vi "Read Page Orientaion V2.vi"(0 "PDF Report IN":refnum<class "PDF Report Class.lvclass">, 5 "PdfReader ref":refnum<k24>, 7 "PdfReader page number":i32=-1, 9 "Page (points)":T2={"Start at page"=1, "Page Size"=0, "Orientation"=enum."Landscape", "widht"=792.0, "height"=72.0, "Margin left"=72.0, "Margin right"=72.0, "Margin top"=72.0, "Margin bottom"=72.0, "X0"=0.0, "X1"=612.0, "Y0"=0.0, "Y1"=792.0} {"Page Size" items=["Custom", "LETTER", "NOTE", "LEGAL", "TABLOID", "EXECUTIVE", "POSTCARD", "A0", "A1", "A2", "A3", "A4", "A5", "A6", "A7", "A8", "A9", "A10", "B0", "B1", "B2", "B3", "B4", "B5", "B6", "B7", "B8", "B9", "B10", "ARCH_E", "ARCH_D", "ARCH_C", "ARCH_B", "ARCH_A", "FLSA", "FLSE", "HALFLETTER", "_11X17", "ID_1", "ID_2", "ID_3", "LEDGER", "CROWN_QUARTO", "LARGE_CROWN_QUARTO", "DEMY_QUARTO", "ROYAL_QUARTO", "CROWN_OCTAVO", "LARGE_CROWN_OCTAVO", "DEMY_OCTAVO", "ROYAL_OCTAVO", "SMALL_PAPERBACK", "PENGUIN_SMALL_PAPERBACK", "PENGUIN_LARGE_PAPERBACK"]}, 11 "error in (no error)":errorcluster) -> (4 "PDF Report OUT":refnum<class "PDF Report Class.lvclass">, 6 "PdfReader ref duplicate":refnum<k24>, 10 "Orientation":T1, 15 "error out":errorcluster)   [LabVIEW 2019, in "Exaprom PDF.lvlib"]
doc: "Version 1.1\nDeveloped by Jean-Marc Simard\nCopyright © 2012, Exaprom Inc.\nAll rights reserved.\nLicense: BSD\n\nWith iTextSharp 4.1.6 (http://itextsharp.sourceforge.net)\nunder Mozilla Public License Version 1.1\n(http://www.mozilla.org/MPL/MPL-1.1.html)"
uses:
  C:/work/niobrara_lv/labview pdf writer fixing/DLL/itextsharp.dll
  DLL/itextsharp.dll
  Controls/Page Controls/Page dimensions.ctl
  Controls/Page Controls/Page Orientation.ctl
  LV Class/PDF Report Class/PDF Report Class.lvclass
  Controls/Page Controls/Page setup.ctl
  Controls/Page Controls/Page Layout Custom.ctl
  Controls/Page Controls/Page margins.ctl
  Exaprom PDF.lvlib
  Controls/Page Controls/Page size.ctl
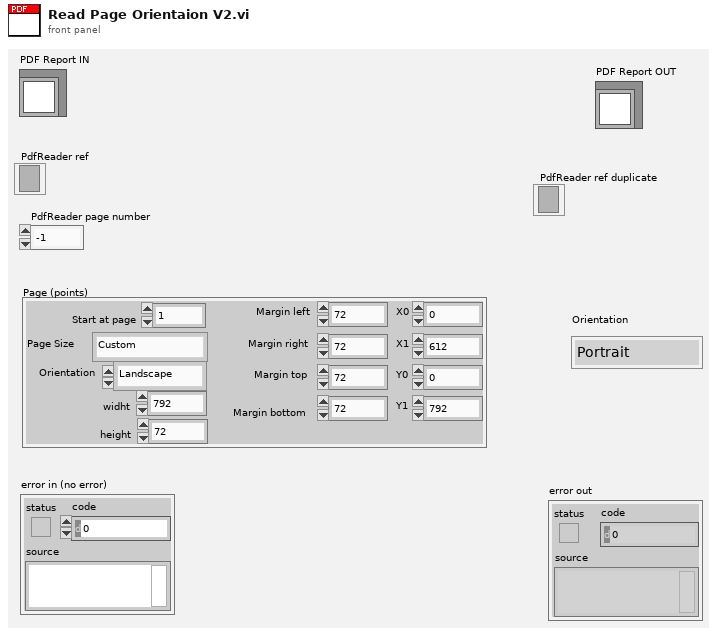
[diagram p1: front panel]
types:
  T1 = typedef "Exaprom PDF.lvlib/Page Orientation.ctl" = enum16{"Portrait", "Landscape"}
  T2 = typedef "Exaprom PDF.lvlib/Page dimensions.ctl" = cluster{"Start at page":i32, "Page Size":T3, "Orientation":T1, "widht":sgl, "height":sgl, "Margin left":sgl, "Margin right":sgl, "Margin top":sgl, "Margin bottom":sgl, "X0":sgl, "X1":sgl, "Y0":sgl, "Y1":sgl}
  T3 = typedef "Exaprom PDF.lvlib/Page size.ctl" = i32
  T4 = typedef "Exaprom PDF.lvlib/Page setup.ctl" = cluster{"Page Size":T3, "Orientation":T1, "Custom Size":T5, "Margins":T6}
  T5 = typedef "Exaprom PDF.lvlib/Page Layout Custom.ctl" = cluster{"Width":sgl, "Height":sgl}
  T6 = typedef "Exaprom PDF.lvlib/Page margins.ctl" = cluster{"Left":sgl, "Right":sgl, "Top":sgl, "Bottom":sgl}
  T7 = typedef "Exaprom PDF.lvlib/Unit.ctl" = enum16{"inch", "mm"}
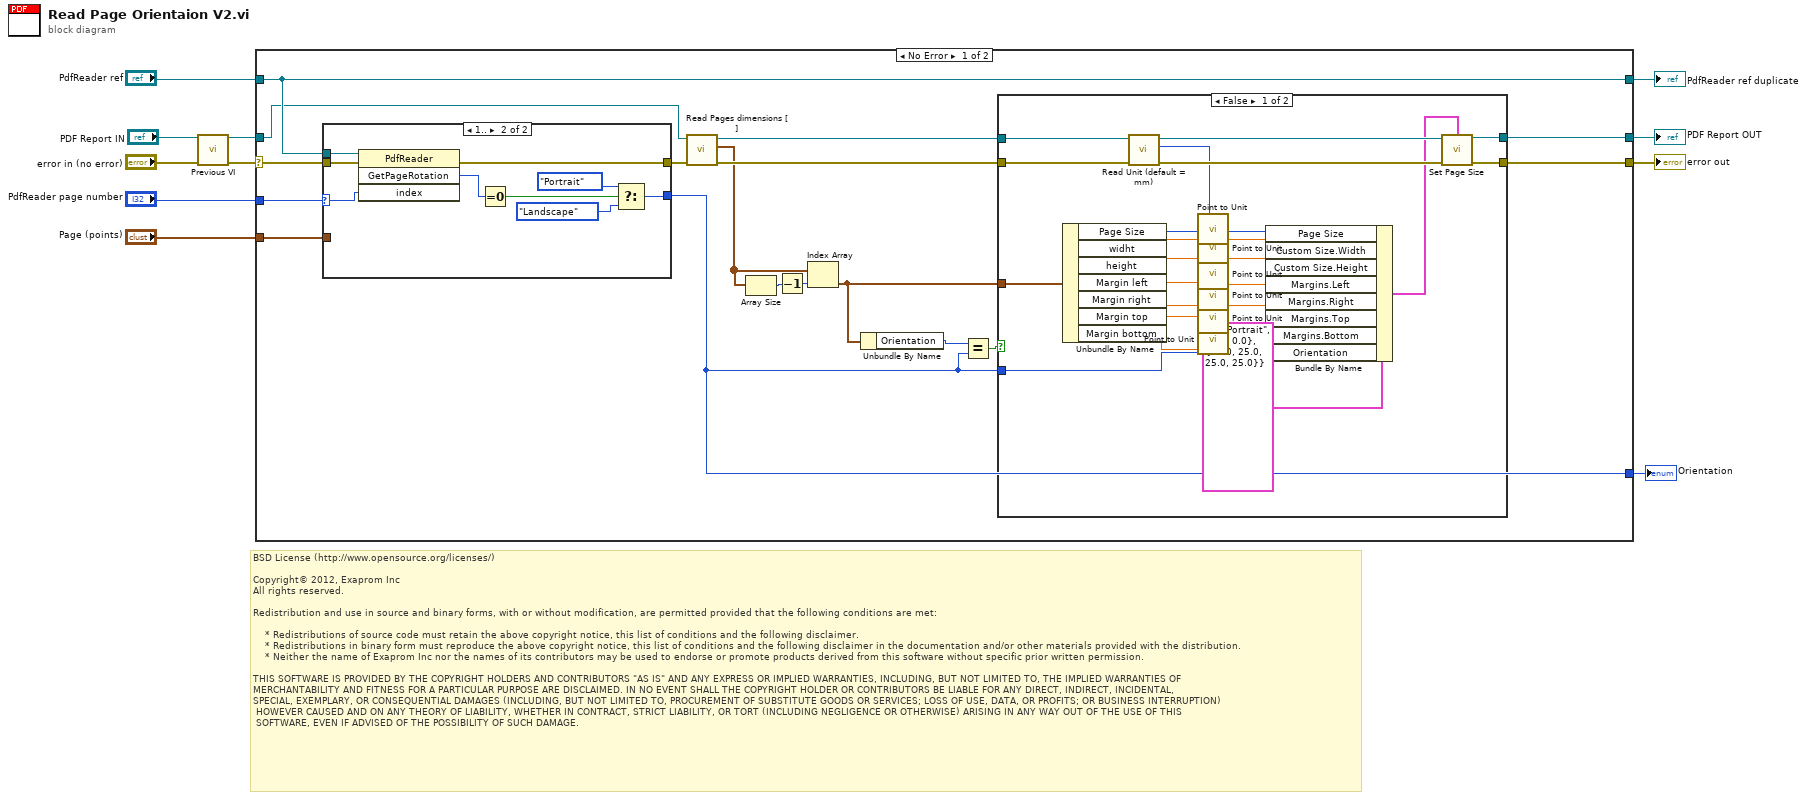
[diagram p0: block diagram]
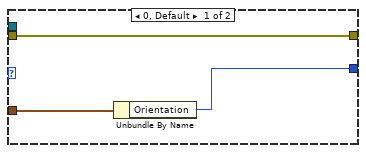
[diagram p2: hidden frame]
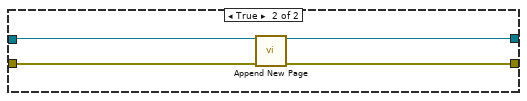
[diagram p3: hidden frame]
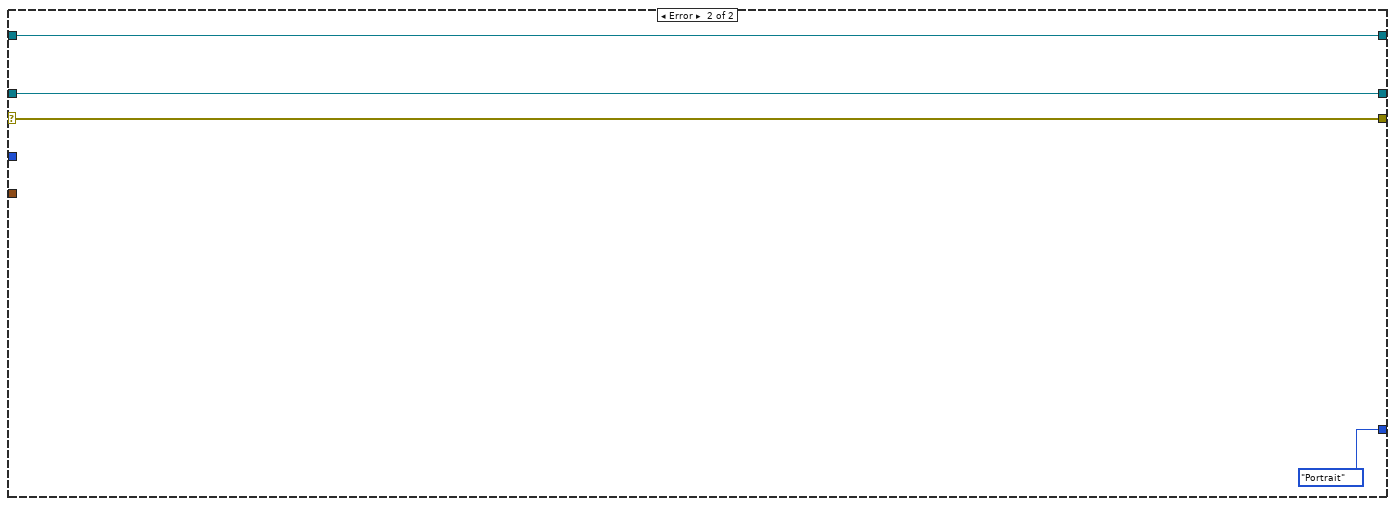
[diagram p4: hidden frame]
diagram:
  # "BSD License (http://www.opensource.org/licenses/)\n\nCopyright© 2012, Exaprom Inc\nAll rights reserved.\n\nRedistribution and use in source and binary forms, with or without modification, are permitted provided that the following conditions are met:\n\n    * Redistributions of source code must retain the above copyright notice, this list of conditions and the following disclaimer.\n    * Redistributions in binary form must reproduce the above copyright notice, this list of conditions and the following disclaimer in the documentation and/or other materials provided with the distribution.\n    * Neither the name of Exaprom Inc nor the names of its contributors may be used to endorse or promote products derived from this software without specific prior written permission.\n\nTHIS SOFTWARE IS PROVIDED BY THE COPYRIGHT HOLDERS AND CONTRIBUTORS \"AS IS\" AND ANY EXPRESS OR IMPLIED WARRANTIES, INCLUDING, BUT NOT LIMITED TO, THE IMPLIED WARRANTIES OF \nMERCHANTABILITY AND FITNESS FOR A PARTICULAR PURPOSE ARE DISCLAIMED. IN NO EVENT SHALL THE COPYRIGHT HOLDER OR CONTRIBUTORS BE LIABLE FOR ANY DIRECT, INDIRECT, INCIDENTAL,\nSPECIAL, EXEMPLARY, OR CONSEQUENTIAL DAMAGES (INCLUDING, BUT NOT LIMITED TO, PROCUREMENT OF SUBSTITUTE GOODS OR SERVICES; LOSS OF USE, DATA, OR PROFITS; OR BUSINESS INTERRUPTION)\n HOWEVER CAUSED AND ON ANY THEORY OF LIABILITY, WHETHER IN CONTRACT, STRICT LIABILITY, OR TORT (INCLUDING NEGLIGENCE OR OTHERWISE) ARISING IN ANY WAY OUT OF THE USE OF THIS\n SOFTWARE, EVEN IF ADVISED OF THE POSSIBILITY OF SUCH DAMAGE."
  n1 = call "Previous VI.vi"("PDF Report IN"="PDF Report IN", "error in (no error)"="error in (no error)") -> ("PDF Report OUT"=w5:refnum<class "PDF Report Class.lvclass">, "error out"=w2:errorcluster)  [unwired: 12 out]
  n2 = case shown="No Error" w2 {
    selector: w2 -> [w26 w72]
    tunnel: [w23 w72] -> w11
    tunnel: [w16 w71] -> w10
    tunnel: "PdfReader page number" -> [w14 _]
    tunnel: "PdfReader ref" -> [w16 w71]
    tunnel: "Page (points)" -> [w13 _]
    tunnel: w5 -> [w15 w70]
    tunnel: [w22 w70] -> w6
    tunnel: [w12 Page_Orientation."Portrait" ("Orientation")] -> w1
    frame No Error {
      n3 = case shown="1.." w14 {
        selector: w14 -> [_ w37]
        tunnel: w26 -> [w31 w40]
        tunnel: [w31 w39] -> w24
        tunnel: w16 -> [_ w38]
        tunnel: [w29 w32] -> w12
        tunnel: w13 -> [w30 _]
        frame 0, Default {
          n4 = Unbundle By Name(w30) -> ("Orientation"=w29:T1)
        }
        frame 1.. {
          n5 = invoke class="PdfReader" method="GetPageRotation"(reference=w38, error in=w40, "index"=w37) -> (error out=w39:errorcluster, "GetPageRotation"=w33:i32)  [unwired: 1 in, 2 out]
          n6 = Equal To 0?(x=w33) -> (x = 0?=w36:bool)
          n7 = Select(t=Page_Orientation."Portrait" ("Orientation"), s=w36, f=Page_Orientation."Landscape" ("Orientation")) -> (s? t:f=w32:T1)
        }
      }
      n8 = call-dynamic "Read Pages dimensions [ ].vi"("error in (no error)"=w24, "PDF Report Class in"=w15) -> ("error out"=w21:errorcluster, "Pages dimensions [ ]"=w18:T2[], "PDF Report Class out"=w20:refnum<class "PDF Report Class.lvclass">)  [unwired: 6 in, 1 out]
      n9 = Array Size(array=w18) -> (size(s)=w28:i32)
      n10 = Decrement(x=w28) -> (x-1=w27:i32)
      n11 = Index Array(array=w18, index=w27) -> (element=w17:T2)
      n12 = Unbundle By Name(w17) -> ("Orientation"=w19:T1)
      n13 = Equal?(x=w19, y=w12) -> (x = y?=w25:bool)
      n14 = case shown="False" w25 {
        tunnel: w21 -> [w64 w68]
        tunnel: [w63 w67] -> w23
        tunnel: [w62 w65] -> w22
        tunnel: w20 -> [w60 w66]
        tunnel: w17 -> [w58 _]
        tunnel: w12 -> [w41 _]
        frame False {
          n15 = Unbundle By Name(w58) -> ("Page Size"=w43:T3, "widht"=w56:sgl, "height"=w52:sgl, "Margin left"=w54:sgl, "Margin right"=w48:sgl, "Margin top"=w53:sgl, "Margin bottom"=w45:sgl)
          n16 = call-dynamic "Read Unit (default = mm).vi"("error in (no error)"=w64, "PDF Report Class in"=w60) -> ("error out"=w61:errorcluster, "Unit (default = mm)"=w44:T7, "PDF Report Class out"=w59:refnum<class "PDF Report Class.lvclass">)  [unwired: 7 in]
          n17 = call "Point to Unit.vi"("X point"=w56, "Unit (default = mm)"=w44) -> ("X unit"=w55:sgl)  [unwired: 7 in]
          n18 = call "Point to Unit.vi"("X point"=w52, "Unit (default = mm)"=w44) -> ("X unit"=w51:sgl)  [unwired: 7 in]
          n19 = call "Point to Unit.vi"("X point"=w54, "Unit (default = mm)"=w44) -> ("X unit"=w50:sgl)  [unwired: 7 in]
          n20 = call "Point to Unit.vi"("X point"=w48, "Unit (default = mm)"=w44) -> ("X unit"=w49:sgl)  [unwired: 7 in]
          n21 = call "Point to Unit.vi"("X point"=w53, "Unit (default = mm)"=w44) -> ("X unit"=w47:sgl)  [unwired: 7 in]
          n22 = call "Point to Unit.vi"("X point"=w45, "Unit (default = mm)"=w44) -> ("X unit"=w46:sgl)  [unwired: 7 in]
          n23 = Bundle By Name(cluster=T4 {"Page Size"=1, "Orientation"=enum."Portrait", "Custom Size"={"Width"=0.0, "Height"=0.0}, "Margins"={"Left"=25.0, "Right"=25.0, "Top"=25.0, "Bottom"=25.0}} ("Page setup"), "Page Size"=w43, "Custom Size.Width"=w55, "Custom Size.Height"=w51, "Margins.Left"=w50, "Margins.Right"=w49, "Margins.Top"=w47, "Margins.Bottom"=w46, "Orientation"=w41) -> (w42:T4)
          n24 = call "Set Page Size.vi"("PDF Report IN"=w59, "Page setup"=w42, "error in (no error)"=w61) -> ("PDF Report OUT"=w62:refnum<class "PDF Report Class.lvclass">, "error OUT"=w63:errorcluster)  [unwired: 11 in]
        }
        frame True {
          n25 = call "Append New Page.vi"("PDF Report"=w66, "error in (no error)"=w68) -> ("PDF Report duplicate"=w65:refnum<class "PDF Report Class.lvclass">, "error OUT"=w67:errorcluster)  [unwired: 12 in]
        }
      }
    }
    frame Error {
    }
  }
  "error out" <- w11
  "PdfReader ref duplicate" <- w10
  "PDF Report OUT" <- w6
  "Orientation" <- w1
